vi "FTP_RETR.vi"(5 "connection ID":refnum<k5>, 6 "Remote Path":string, 7 "error in":errorcluster) -> (0 "connection ID out":refnum<k5>, 1 "reply string":string, 2 "vi":string, 3 "error out":errorcluster, 4 "Good Reply?":bool)   [LabVIEW 2012]
panel:
  in  "chunk size (4096)":i32=4096
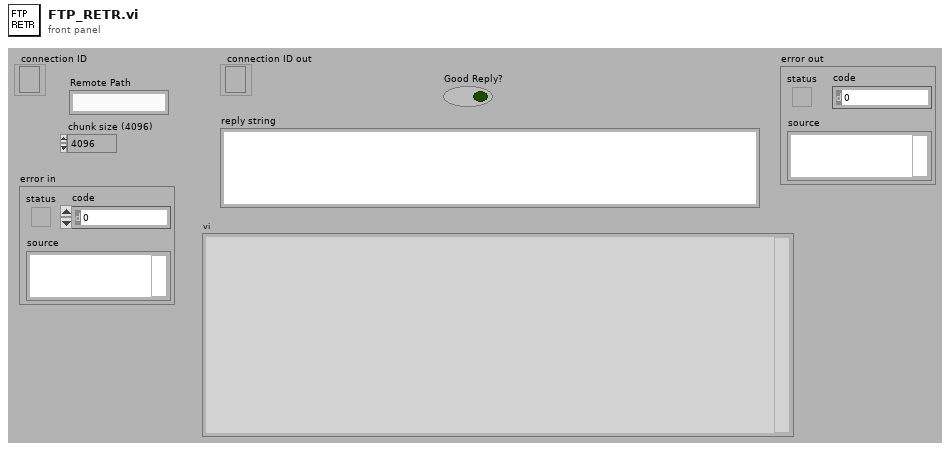
[diagram p1: front panel]
types:
  T1 = enum16{"unknown", "100 + Prelim", "200 + ", "300 + Intermed", "400 - Transient", "500 - Permanent"}
  T2 = cluster{"passive address":string, "passive port":u16}
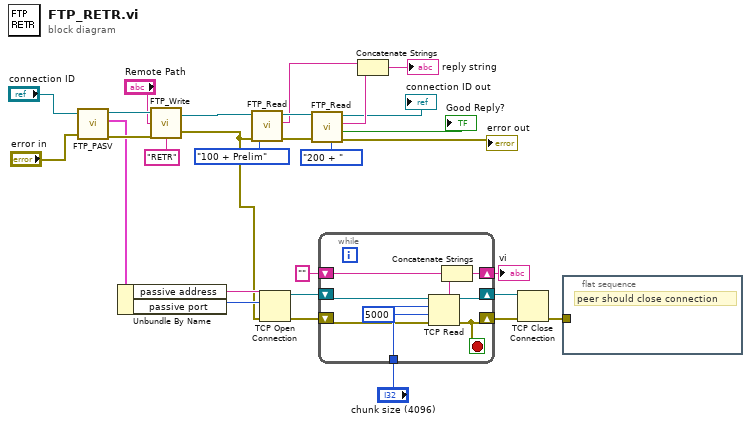
[diagram p0: block diagram]
diagram:
  n1 = call <userlib>:"FTP_PASV.vi"("connection ID"="connection ID", "error in"="error in") -> ("connection ID out"=w24:refnum<k5>, "Passive Port"=w16:T2, "error out"=w23:errorcluster)  [unwired: 2 out]
  n2 = Unbundle By Name(w16) -> ("passive address"=w17:string, "passive port"=w18:u16)
  n3 = call <userlib>:"FTP_Write.vi"("Cmd"="RETR", "error in"=w23, "data"="Remote Path", "connection ID in"=w24) -> ("error out"=w11:errorcluster, "connection ID out"=w27:refnum<k5>)
  n4 = call <userlib>:"FTP_Read.vi"("error In"=w11, "expected class"=T1."100 + Prelim", "connection ID"=w27) -> ("error out"=w7:errorcluster, "reply string"=w6:string, "connection ID out"=w8:refnum<k5>)  [unwired: 2 out]
  n5 = TCP Open Connection(address=w17, remote port or service name=w18, error in (no error)=w11) -> (connection ID=w19:refnum<k5>, error out=w20:errorcluster)  [unwired: 2 out]
  n6 = call <userlib>:"FTP_Read.vi"("error In"=w7, "expected class"=T1."200 + ", "connection ID"=w8) -> ("error out"=→"error out":errorcluster, "Good Reply?"=→"Good Reply?":bool, "reply string"=w5:string, "connection ID out"=→"connection ID out":refnum<k5>)  [unwired: 1 out]
  n7 = while {
    shift-right: [w34] -> w22
    shift-left: w19 -> [w36]
    shift-right: [w30] -> w21
    shift-left: w20 -> [w35]
    tunnel: "chunk size (4096)" -> [w37]
    shift-right: [w31] -> w12
    shift-left: "" -> [w33]
    stop <- w30 stop-if-true
    n8 = TCP Read(connection ID=w36, bytes to read=w37, error in (no error)=w35, 9:5000 ("timeout ms (25000)")) -> (connection ID out=w34:refnum<k5>, data out=w32:string, error out=w30:errorcluster)  [unwired: 1 out]
    n9 = Concatenate Strings(w33, w32) -> (w31:string)
  }
  "vi" <- w12
  n10 = Concatenate Strings(w6, w5) -> (→"reply string":string)
  n11 = TCP Close Connection(connection ID=w22, error in (no error)=w21) -> (error out=w13:errorcluster)  [unwired: 2 out]
  n12 = flat-sequence {
    tunnel: w13 -> [_]
    frame #0 {
      # "peer should close connection"
    }
  }
